vi "Perform Action Core.vi"(8 "error in (no error)":errorcluster, 11 "NI DMM in":refnum<class "NI DMM.lvclass">) -> (0 "error out":errorcluster, 3 "NI DMM out":refnum<class "NI DMM.lvclass">)   [LabVIEW 2023, in "NI DMM.lvlib" / "NI DMM.lvclass"]
uses:
  NI DMM.lvclass
  NI DMM.lvclass/NI DMM.ctl
  Device/Device/Device.lvclass
  <instrlib>/niDMM/nidmm.llb/niDMM Fetch Waveform (waveform data).vi
  D:/2_GitHub/LabVIEW-Device/Device/Device/Device.lvclass
  C:/Program Files (x86)/National Instruments/LabVIEW 2023/vi.lib/ActorFramework/Actor/Actor.lvclass
  D:/2_GitHub/LabVIEW-Device/Device Driver/NI DMM/NI DMM/NI DMM.lvclass
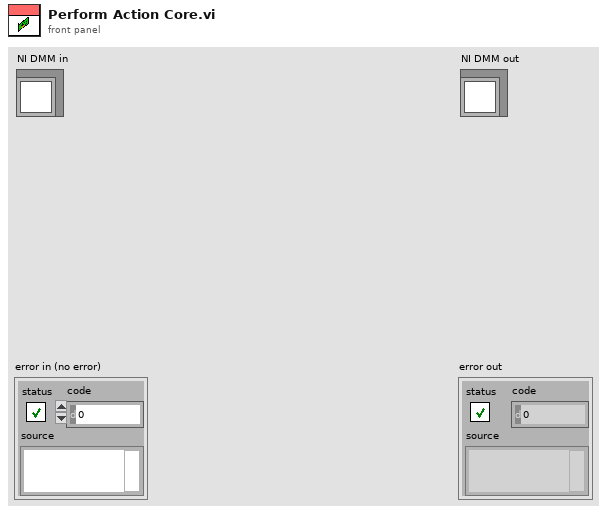
[diagram p1: front panel]
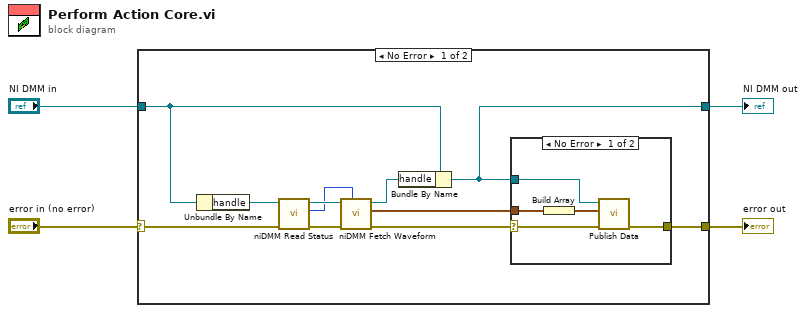
[diagram p0: block diagram]
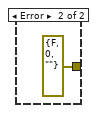
[diagram p2: hidden frame]
diagram:
  n1 = case shown="No Error" "error in (no error)" {
    selector: "error in (no error)" -> [w15 w23]
    tunnel: "NI DMM in" -> [w9 w22]
    tunnel: [w5 w23] -> w2
    tunnel: [w7 w22] -> w1
    frame No Error {
      n2 = Unbundle By Name(w9) -> ("handle"=w14:refnum<k15>)
      n3 = call <instrlib>:"niDMM Read Status.vi"("error in (no error)"=w15, "instrument handle"=w14) -> ("error out"=w12:errorcluster, "Backlog"=w11:i32, "instrument handle out"=w13:refnum<k15>)  [unwired: 6 in, 1 out]
      n4 = call-poly <instrlib>:"niDMM Fetch Waveform.vi"("Number To Fetch"=w11, "error in (no error)"=w12, "instrument handle"=w13) -> ("error out"=w10:errorcluster, "Waveform Data"=w6:waveform(dbl), "instrument handle out"=w8:refnum<k15>)  [unwired: 5 in, 1 out]
      n5 = Bundle By Name(cluster=w9, "handle"=w8) -> (w7:refnum<class "NI DMM.lvclass">)
      n6 = case shown="No Error" w10 {
        selector: w10 -> [w20 _]
        tunnel: w7 -> [w17 _]
        tunnel: w6 -> [w19 _]
        tunnel: [w16 errorcluster {"status"=FALSE, "code"=0, "source"=""} ("error out")] -> w5
        frame No Error {
          n7 = Build Array(w19) -> (w18:waveform(dbl)[])
          n8 = call "Publish Data.vi"("error in (no error)"=w20, "waveform"=w18, "Device in"=w17) -> ("error out"=w16:errorcluster)  [unwired: 7 in, 1 out]
        }
        frame Error {
        }
      }
    }
    frame Error {
    }
  }
  "error out" <- w2
  "NI DMM out" <- w1
